vi "CheckReceiverState.vi"(8 "error in (no error)":errorcluster, 11 "object in":refnum<class "PrimaryAttackerRole.lvclass">) -> (0 "error out":errorcluster, 2 "pass":bool=TRUE, 3 "object out":refnum<class "PrimaryAttackerRole.lvclass">)   [LabVIEW 2023, in "PrimaryAttackerRole.lvclass"]
uses:
  PrimaryAttackerRole.lvclass
  PrimaryAttackerRole.lvclass/PrimaryAttackerRole.ctl
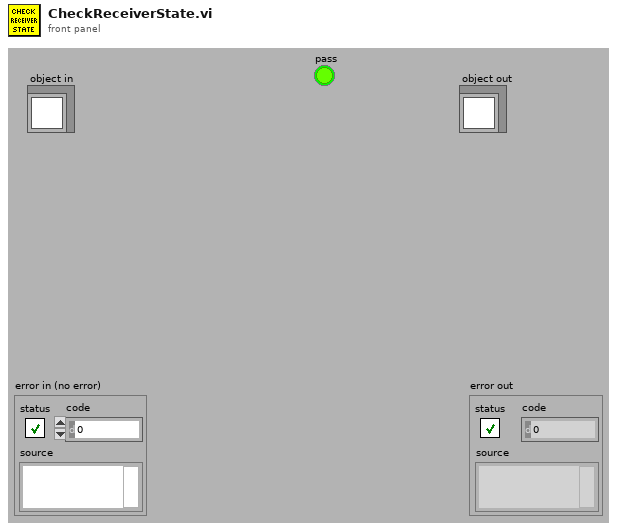
[diagram p1: front panel]
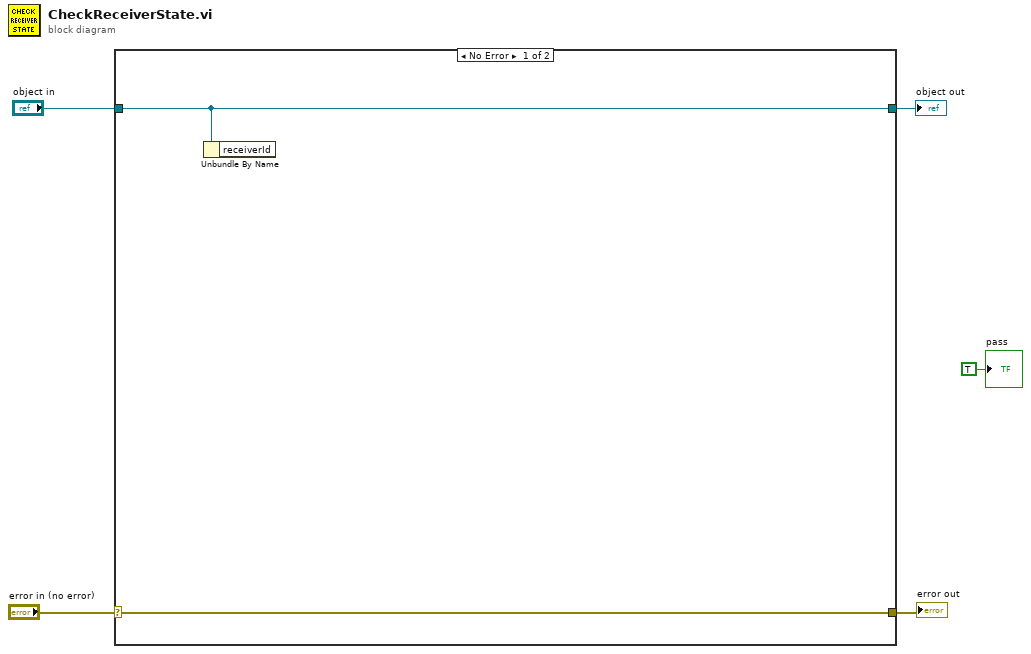
[diagram p0: block diagram]
diagram:
  n1 = case shown="No Error" "error in (no error)" {
    selector: "error in (no error)" -> [w7 w9]
    tunnel: [w7 w9] -> w4
    tunnel: [w6 w8] -> w2
    tunnel: "object in" -> [w6 w8]
    frame No Error {
      n2 = Unbundle By Name(w6) -> ()  [unwired: 1 out]
    }
    frame Error {
    }
  }
  "error out" <- w4
  "object out" <- w2
  "pass" <- TRUE ("pass")
